vi "LVCAM Destroy Self.vi"(11 "Process in":refnum<class "Process.lvclass">) -> (0 "error out":errorcluster, 1 "Destroyed Self?":bool, 3 "Process out":refnum<class "Process.lvclass">)   [LabVIEW 2021, in "Process.lvlib" / "Process.lvclass"]
uses:
  Process.lvclass
  Process.lvclass/Process.ctl
  LVCAM/LVCAM/LVCAM/LVCAM.lvclass
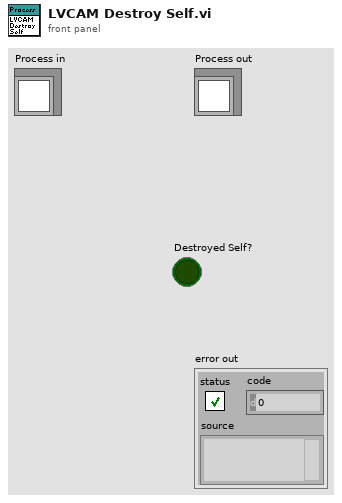
[diagram p1: front panel]
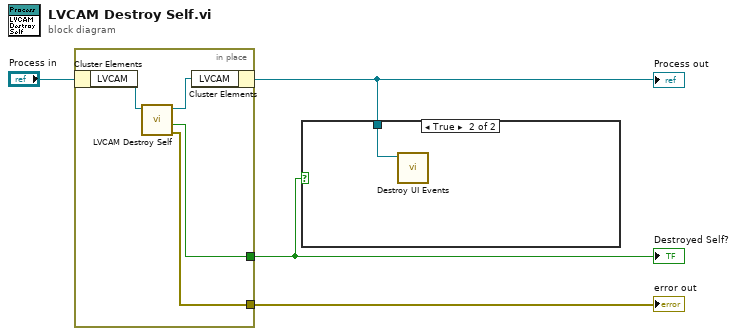
[diagram p0: block diagram]
diagram:
  n1 = in-place {
    in-place-border: [w6] -> w2
    in-place-border: [w5] -> w3
    n2 = in-place-cluster #1("Process in") -> ("LVCAM"=w8:refnum<class "LVCAM.lvclass">)
    n3 = call-dynamic "LVCAM Destroy Self.vi"("LVCAM Destroy Self in"=w8) -> ("error out"=w5:errorcluster, "Destroyed Self?"=w6:bool, "LVCAM Destroy Self out"=w7:refnum<class "LVCAM.lvclass">)  [unwired: 8 in]
    n4 = in-place-cluster #1("LVCAM"=w7) -> (w1:refnum<class "Process.lvclass">)
  }
  "error out" <- w3
  "Process out" <- w1
  "Destroyed Self?" <- w2
  n5 = case shown="True" w2 {
    tunnel: w1 -> [_ w9]
    frame False {
    }
    frame True {
      n6 = call "Destroy UI Events.vi"("Process in"=w9) -> ()  [unwired: 11 in]
    }
  }
